vi "Fiducial Autofocus.vi"(6 "X, Y pixel stride":dbl[](array[numeric])=[1520.0, 2160.0], 8 "Image":T1(plugin-control), 9 "Loop count":dbl=1.0, 11 "Gantry In":refnum<k24>) -> (3 "Gantry Out":refnum<k24>)   [LabVIEW 2021]
uses:
  C:/Program Files (x86)/Aerotech/A3200/LabVIEW/2010/Bin/Aerotech.A3200.dll
  Program Files (x86)/Aerotech/A3200/LabVIEW/2010/Bin/Aerotech.A3200.dll
  Classes/Controller/Motion/A3200/A3200.lvclass
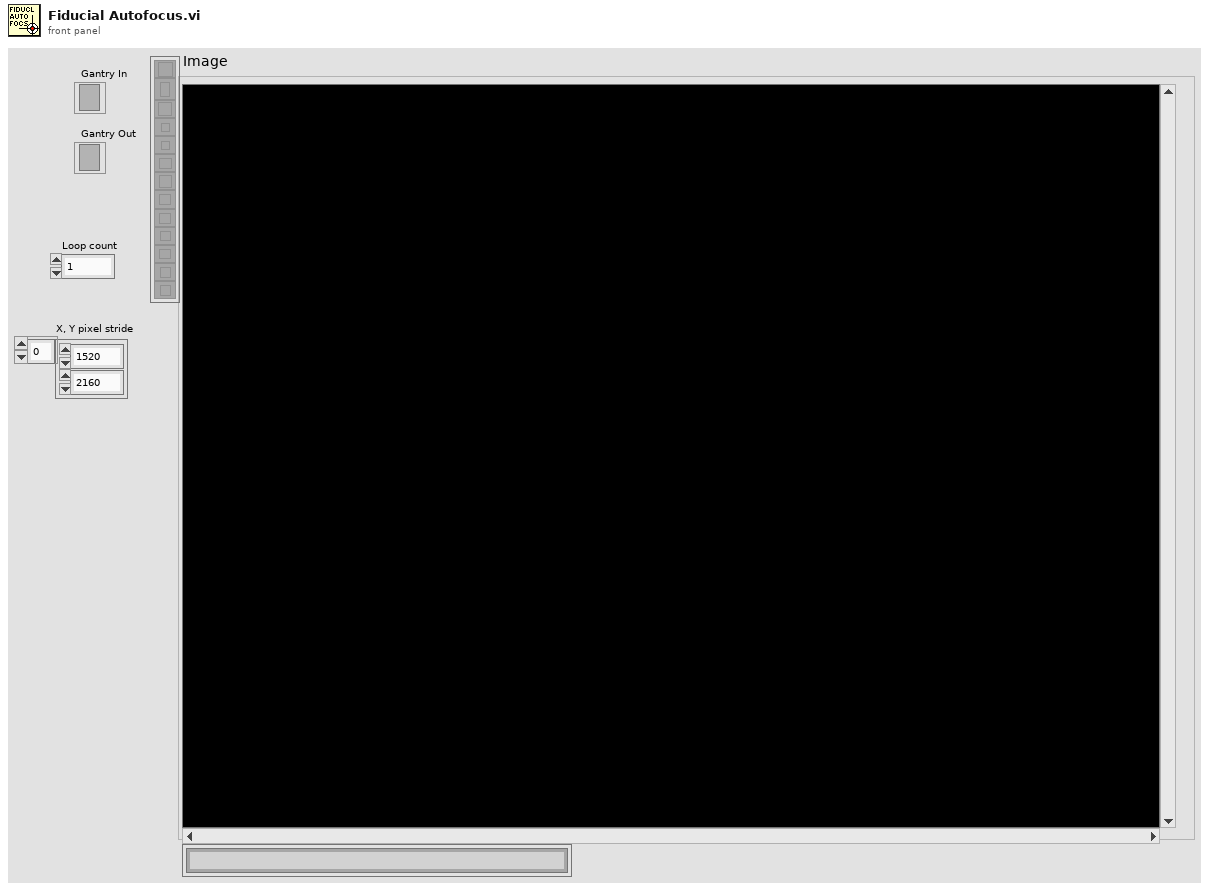
[diagram p1: front panel]
types:
  T1 = typedef "IMAQ Image.ctl" = refnum<image>
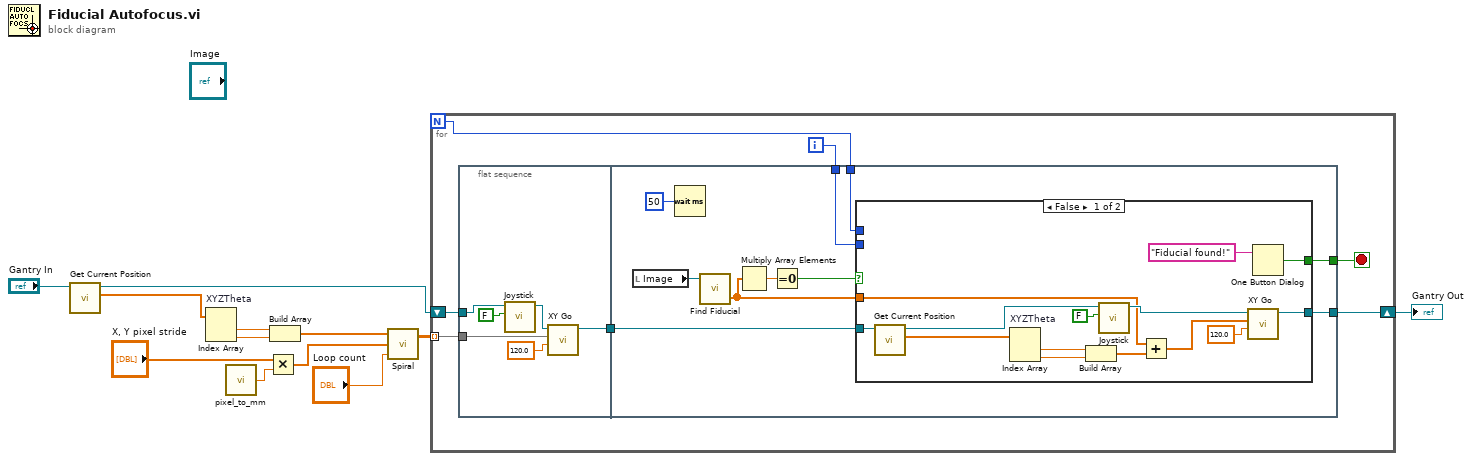
[diagram p0: block diagram]
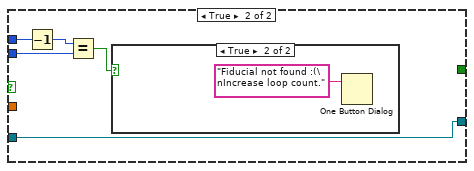
[diagram p2: hidden frame]
diagram:
  n1 = call "Get Current Position.vi"("Gantry In"="Gantry In") -> ("XYZTheta Out"=w11:dbl[], "Gantry Out"=w12:refnum<k24>)  [unwired: 8 in, 1 out]
  n2 = Index Array "XYZTheta"(array=w11) -> (element #1=w10:dbl, element #2=w9:dbl)  [unwired: 2 in]
  n3 = call "pixel_to_mm.vi"() -> ("mm/pixel"=w6:dbl)  [unwired: 2 in]
  n4 = Multiply(x="X, Y pixel stride", y=w6) -> (x*y=w5:dbl[])
  n5 = Build Array(w10, w9) -> (w8:dbl[])
  n6 = call "Spiral.vi"("Loop count"="Loop count", "X, Y stride (mm)"=w5, "XY center (mm)"=w8) -> ("Spiral coordinates"=w3:dbl[][])  [unwired: 1 in]
  n7 = for {
    N -> [w15]
    tunnel: w3 -> [w19] mode=indexing
    shift-right: [w17] -> w1
    shift-left: w12 -> [w18]
    i -> [w14]
    stop <- w16 stop-if-true
    n8 = flat-sequence {
      tunnel: [w20] -> w13
      tunnel: w18 -> [w22]
      tunnel: w19 -> [w21]
      tunnel: [w32] -> w17
      tunnel: [w34] -> w16
      tunnel: w15 -> [w31]
      tunnel: w14 -> [w30]
      tunnel: w13 -> [w29]
      frame #0 {
        n9 = call "Joystick.vi"("Joystick"=FALSE, "Gantry In"=w22) -> ("Gantry Out"=w25:refnum<k24>)  [unwired: 8 in, 1 out]
        n10 = call "XY Go.vi"("Speed"=120.0, "XY In"=w21, "Gantry In"=w25) -> ("Gantry Out"=w20:refnum<k24>)  [unwired: 6 in, 2 out]
      }
      frame #1 {
        n11 = local read "Image"() -> (w35:T1)
        n12 = Wait (ms)(milliseconds to wait=u32 50) -> ()  [unwired: 1 out]
        n13 = call "Find Fiducial.vi"("Image"=w35) -> ("Move by (mm)"=w33:dbl[])  [unwired: 3 in]
        n14 = Multiply Array Elements(1:w33) -> (0:w27:dbl)
        n15 = Equal To 0?(x=w27) -> (x = 0?=w26:bool)
        n16 = case shown="False" w26 {
          tunnel: [w39 _] -> w34
          tunnel: w33 -> [w38 _]
          tunnel: [w37 w50] -> w32
          tunnel: w31 -> [_ w52]
          tunnel: w30 -> [_ w51]
          tunnel: w29 -> [w36 w50]
          frame False {
            n17 = call "Get Current Position.vi"("Gantry In"=w36) -> ("XYZTheta Out"=w44:dbl[], "Gantry Out"=w49:refnum<k24>)  [unwired: 8 in, 1 out]
            n18 = Index Array "XYZTheta"(array=w44) -> (element #1=w45:dbl, element #2=w46:dbl)  [unwired: 2 in]
            n19 = Build Array(w45, w46) -> (w47:dbl[])
            n20 = call "Joystick.vi"("Joystick"=FALSE, "Gantry In"=w49) -> ("Gantry Out"=w43:refnum<k24>)  [unwired: 8 in, 1 out]
            n21 = Add(x=w38, y=w47) -> (x+y=w48:dbl[])
            n22 = call "XY Go.vi"("Speed"=120.0, "XY In"=w48, "Gantry In"=w43) -> ("Gantry Out"=w37:refnum<k24>)  [unwired: 6 in, 2 out]
            n23 = One Button Dialog(message="Fiducial found!") -> (true=w39:bool)  [unwired: 1 in]
          }
          frame True {
            n24 = Decrement(x=w52) -> (x-1=w54:i32)
            n25 = Equal?(x=w54, y=w51) -> (x = y?=w53:bool)
            n26 = case shown="True" w53 {
              frame False {
              }
              frame True {
                n27 = One Button Dialog(message="Fiducial not found :(\nIncrease loop count.") -> ()  [unwired: 1 in, 1 out]
              }
            }
          }
        }
      }
    }
  }
  "Gantry Out" <- w1
